vi "Init.vi"(6 "Timeout, s":dbl=30.0, 8 "error in (no error)":errorcluster, 9 "VXM ACK que":T1, 10 "VXM Svc que":T1, 11 "Standalone":bool=TRUE) -> (0 "error out":errorcluster, 3 "MotionComm out":refnum<class "MotionComm.lvclass">)   [LabVIEW 2018, in "MotionComm.lvclass"]
uses:
  MotionComm.lvclass
  Support/MessageQue/MessageQue.ctl
  Support/MessageQue/MessageCluster.ctl
  MotionComm.lvclass/MotionComm.ctl
  Support/MessageQue/MessageQue.lvlib
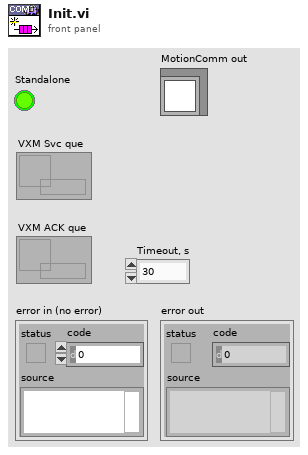
[diagram p1: front panel]
types:
  T1 = typedef "MessageQue.lvlib/MessageQue.ctl" = refnum<queue>
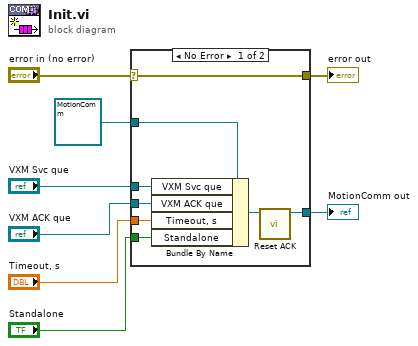
[diagram p0: block diagram]
diagram:
  n1 = case shown="No Error" "error in (no error)" {
    selector: "error in (no error)" -> [w15 w18]
    tunnel: [w15 w18] -> w7
    tunnel: [w10 w17] -> w5
    tunnel: refnum<class "MotionComm.lvclass"> refnum ("MotionComm in") -> [w16 w17]
    tunnel: "VXM Svc que" -> [w14 _]
    tunnel: "VXM ACK que" -> [w13 _]
    tunnel: "Timeout, s" -> [w12 _]
    tunnel: "Standalone" -> [w11 _]
    frame No Error {
      n2 = Bundle By Name(cluster=w16, "VXM Svc que"=w14, "VXM ACK que"=w13, "Timeout, s"=w12, "Standalone"=w11) -> (w9:refnum<class "MotionComm.lvclass">)
      n3 = call "Reset ACK.vi"("MotionComm in"=w9) -> ("MotionComm out"=w10:refnum<class "MotionComm.lvclass">)  [unwired: 9 in, 1 out]
    }
    frame Error {
    }
  }
  "error out" <- w7
  "MotionComm out" <- w5
